vi "plus generate test.vi"(8 "error in (no error)":errorcluster, 9 "Pulse Shaping Filter Coefficients":dbl[](graph), 10 "Samples Per Symbol (16)":i32=16, 11 "Symbols":cdb[](array[numeric]) format="%.2f") -> (0 "error out":errorcluster)   [LabVIEW 2010]
uses:
  <vilib>/measure/masml.llb/ma_sml_Interpolation by Zero Insert (complex input).vi
  <vilib>/Analysis/3filter.llb/IIR Filter (CDB).vi
  <vilib>/measure/NI_MAPro.lvlib
  <vilib>/Analysis/NI_AALBase.lvlib
  <vilib>/addons/Modulation/niAMT.lvlib
panel:
  out "大小 4":i32
  out "大小 3":i32
  out "大小 2":i32
  in  "flush buffers? (F)":bool
  out "大小":i32
  out "Symbols 2":cdb[](array[numeric])
  out "Symbols 3":dbl[](graph)
  out "Symbols 4":dbl[](graph)
  out "Filtered Samples":dbl[](graph)
  in  "Reset? (T)":bool=TRUE
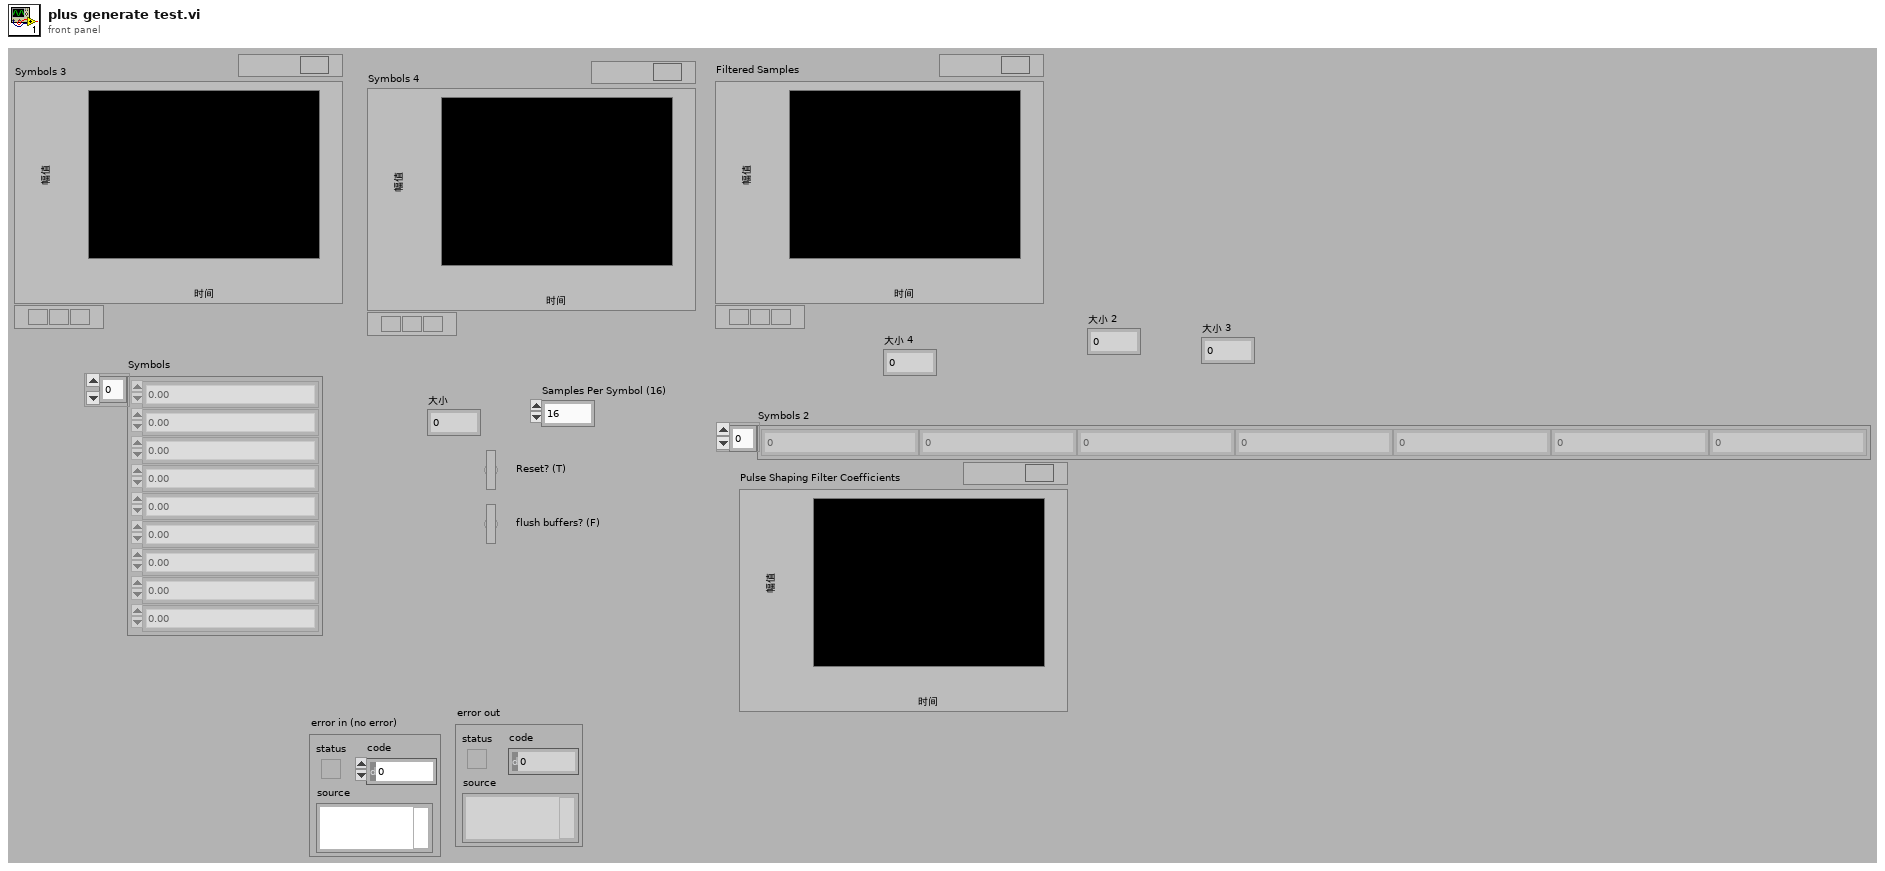
[diagram p1: front panel]
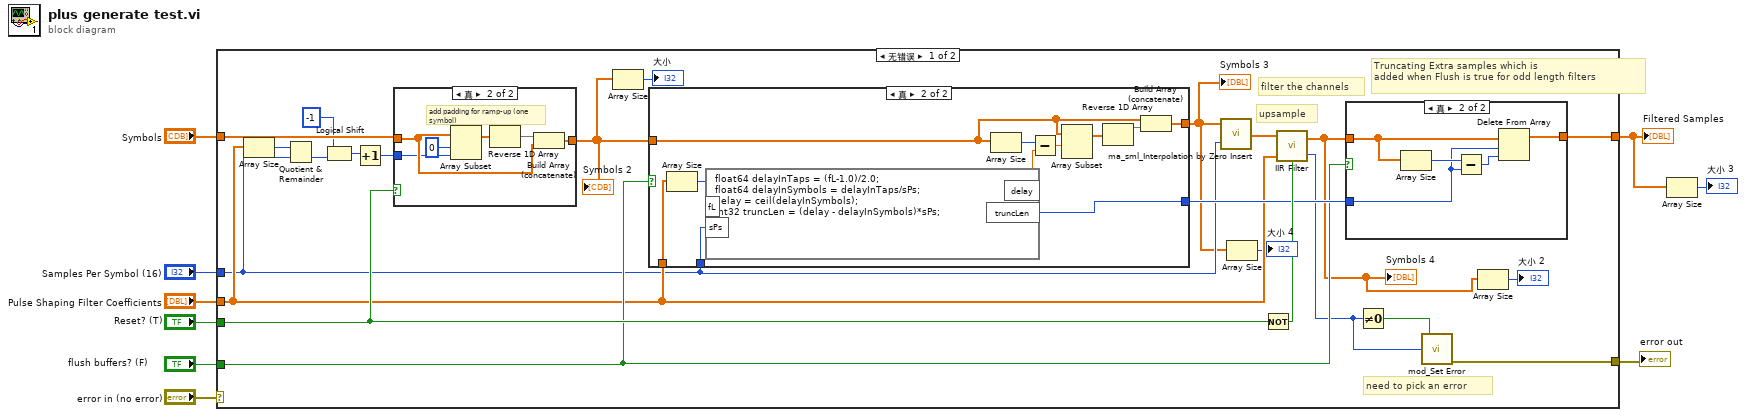
[diagram p0: block diagram]
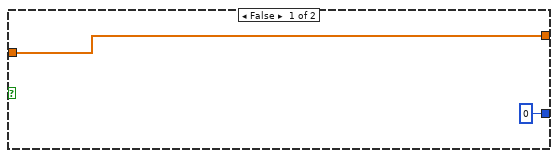
[diagram p3: hidden frame]
diagram:
  n1 = case shown="无错误" "error in (no error)" {
    selector: "error in (no error)" -> [_ w60]
    tunnel: "Pulse Shaping Filter Coefficients" -> [w22 _]
    tunnel: "Symbols" -> [w30 w59]
    tunnel: "Samples Per Symbol (16)" -> [w20 _]
    tunnel: "Reset? (T)" -> [w29 _]
    tunnel: [w28 w59] -> w1
    tunnel: [w31 w60] -> w4
    tunnel: "flush buffers? (F)" -> [w26 _]
    frame No Error {
      # "Truncating Extra samples which is               \nadded when Flush is true for odd length filters"
      # "filter the channels"
      # "upsample"
      # "need to pick an error"
      n2 = Array Size(array=w22) -> (size(s)=w21:i32)
      n3 = Quotient & Remainder(x=w21, y=w20) -> (floor(x/y)=w19:i32)  [unwired: 1 out]
      n4 = Logical Shift(y=i8 -1, x=w19) -> (x << y=w17:i32)
      n5 = Increment(x=w17) -> (x+1=w16:i32)
      n6 = case shown="真" w29 {
        tunnel: w30 -> [w52 w56]
        tunnel: [w52 w55] -> w15
        tunnel: w16 -> [_ w54]
        frame False {
        }
        frame True {
          # "add padding for ramp-up (one symbol)"
          n7 = Array Subset(array=w56, index=0, length=w54) -> (w57:cdb[])
          n8 = Reverse 1D Array(array=w57) -> (reversed array=w53:cdb[])
          n9 = Build Array (concatenate)(w53, w56) -> (w55:cdb[])
        }
      }
      "Symbols 2" <- w15
      n10 = Array Size(array=w15) -> (size(s)=→"大小":i32)
      n11 = case shown="真" w26 {
        tunnel: w22 -> [_ w51]
        tunnel: w20 -> [_ w44]
        tunnel: w15 -> [w40 w47]
        tunnel: [w40 w48] -> w10
        tunnel: [0 w42] -> w27
        frame False {
        }
        frame True {
          n12 = Array Size(array=w51) -> (size(s)=w45:i32)
          n13 = formula code="float64 delayInTaps = (fL-1.0)/2.0;\nfloat64 delayInSymbols = delayInTaps/sPs;\ndelay = ceil(delayInSymbols);\nint32 truncLen = (delay - delayInSymbols)*sPs;"("fL"=w45, "sPs"=w44) -> ("delay"=w43:dbl, "truncLen"=w42:i32)
          n14 = Array Size(array=w47) -> (size(s)=w49:i32)
          n15 = Subtract(x=w49, y=w43) -> (x-y=w50:dbl)
          n16 = Array Subset(array=w47, index=w50) -> (w46:cdb[])  [unwired: 1 in]
          n17 = Reverse 1D Array(array=w46) -> (reversed array=w41:cdb[])
          n18 = Build Array (concatenate)(w47, w41) -> (w48:cdb[])
        }
      }
      "Symbols 3" <- w10
      n19 = call-poly <vilib>:"ma_sml_Interpolation by Zero Insert.vi"("L"=w20, "x"=w10) -> ("y"=w25:cdb[])
      n20 = Array Size(array=w10) -> (size(s)=→"大小 4":i32)
      n21 = Not(x=w29) -> (.not. x?=w32:bool)
      n22 = call-poly <vilib>:"IIR Filter.vi"("init/cont (init:F)"=w32, "Forward Coefficients"=w22, "X"=w25) -> ("error"=w23:i32, "Filtered X"=w12:cdb[])  [unwired: 1 in]
      "Symbols 4" <- w12
      n23 = case shown="真" w26 {
        tunnel: [w33 w38] -> w28
        tunnel: w27 -> [_ w35]
        tunnel: w12 -> [w33 w34]
        frame False {
        }
        frame True {
          n24 = Array Size(array=w34) -> (size(s)=w37:i32)
          n25 = Subtract(x=w37, y=w35) -> (x-y=w36:i32)
          n26 = Delete From Array(array=w34, length=w35, index=w36) -> (array with subset deleted=w38:cdb[])  [unwired: 1 out]
        }
      }
      n27 = Not Equal To 0?(x=w23) -> (x != 0?=w24:bool)
      n28 = call <vilib>:"mod_Set Error.vi"("code"=w23, "status"=w24) -> ("error out"=w31:errorcluster)  [unwired: 6 out]
      n29 = Array Size(array=w12) -> (size(s)=→"大小 2":i32)
    }
    frame Error {
    }
  }
  "error out" <- w4
  "Filtered Samples" <- w1
  n30 = Array Size(array=w1) -> (size(s)=→"大小 3":i32)
